vi "Flatten.vi"(8 "error in (no error)":errorcluster, 11 "Message in":refnum<class "Message.lvclass">) -> (0 "error out":errorcluster, 2 "Buffer":u8[](array[numeric]) format="%.0x", 3 "Message out":refnum<class "Message.lvclass">)   [LabVIEW 2020, in "LV-Proto.lvlib" / "Message.lvclass"]
uses:
  Message.lvclass
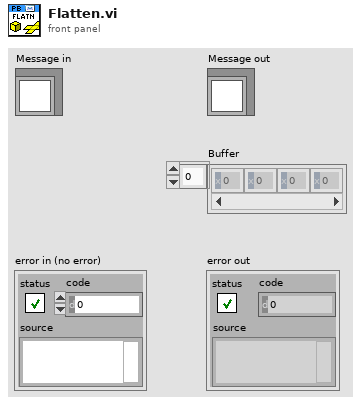
[diagram p1: front panel]
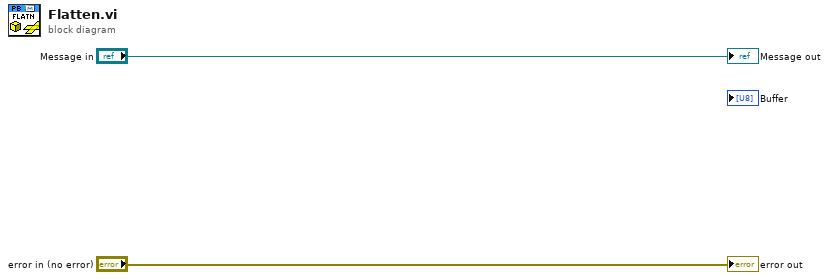
[diagram p0: block diagram]
diagram:
  "error out" <- "error in (no error)"
  "Message out" <- "Message in"
